vi "Init.vi"(5 "Stop User Event in":refnum<user-event>, 7 "Ref FP in":refnum<vi>, 8 "error in (no error)":errorcluster, 9 "Period (ms) in":i64=15, 11 "Mouse Controller in":refnum<class "Mouse.lvclass">) -> (0 "error out":errorcluster, 3 "Mouse Controller out":refnum<class "Mouse.lvclass">)   [LabVIEW 2024, in "Mouse.lvclass"]
doc: "MIT Licence\nCopyright (c) 2024 David Grollier"
uses:
  Mouse.lvclass
  Mouse.lvclass/Mouse.ctl
  Input Device.lvclass
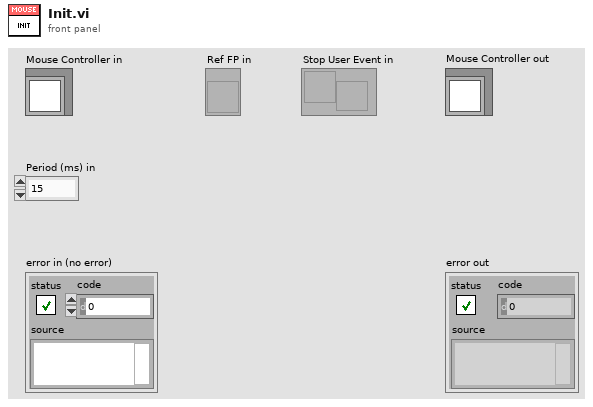
[diagram p1: front panel]
types:
  T1 = typedef "LVRectTypeDef.ctl" = cluster{"Left":i16, "Top":i16, "Right":i16, "Bottom":i16}
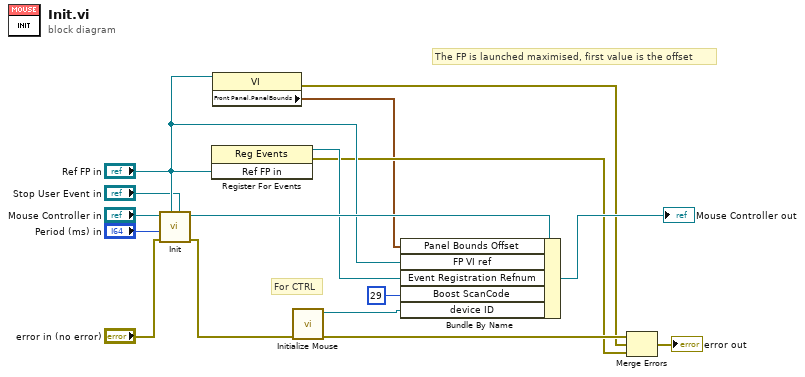
[diagram p0: block diagram]
diagram:
  # "The FP is launched maximised, first value is the offset"
  # "For CTRL"
  n1 = call-parent "Init.vi"("Stop User Event in"="Stop User Event in", "Ref FP in"="Ref FP in", "error in (no error)"="error in (no error)", "Period (ms) in"="Period (ms) in", "Input Device in"="Mouse Controller in") -> ("error out"=w11:errorcluster, "Input Device out"=w13:refnum<class "Mouse.lvclass">)  [unwired: 5 in]
  n2 = register-events("Ref FP in") -> (reference out=w9:refnum<event-registration>, error out=w4:errorcluster)  [unwired: 2 in]
  n3 = property class="VI"(reference="Ref FP in") -> (error out=w5:errorcluster, "Front Panel.PanelBounds"=w2:T1)  [unwired: 1 in, 1 out]
  n4 = call <vilib>:"Initialize Mouse.vi"("error in (no error)"=w11) -> ("error out"=w6:errorcluster, "device ID"=w14:refnum<k1>)  [unwired: 9 in]
  n5 = Bundle By Name(cluster=w13, "Panel Bounds Offset"=w2, "FP VI ref"="Ref FP in", "Event Registration Refnum"=w9, "Boost ScanCode"=i16 29, "device ID"=w14) -> (→"Mouse Controller out":refnum<class "Mouse.lvclass">)
  n6 = Merge Errors(w6, w5, w4) -> (→"error out":errorcluster)
